vi "read pre-execution timing tags.vi"(8 "error in":errorcluster, 11 "Standard Engine Configuration in":refnum<class "Standard Engine Configuration.lvclass">) -> (0 "error out":errorcluster, 2 "execution timing tags":T1, 3 "Standard Engine Configuration out":refnum<class "Standard Engine Configuration.lvclass">)   [LabVIEW 2013, in "Standard Engine Configuration.lvclass"]
doc: "Returns the timing status tags previously configured by the 'enable timing reporting.vi'."
uses:
  Standard Engine Configuration.lvclass
  execution timing tags.ctl
  Standard Engine Configuration.lvclass/Standard Engine Configuration.ctl
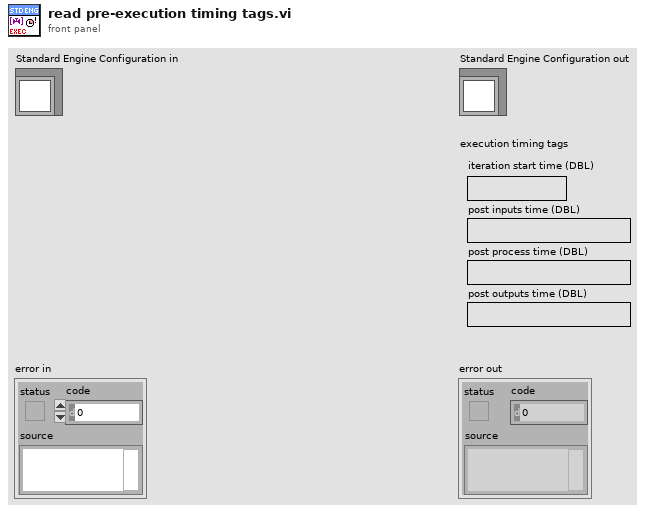
[diagram p1: front panel]
types:
  T1 = typedef "Standard Engine Configuration.lvclass/execution timing tags.ctl" = cluster{"iteration start time (DBL)":string, "post inputs time (DBL)":string, "post process time (DBL)":string, "post outputs time (DBL)":string}
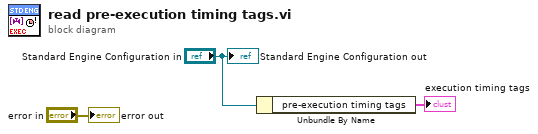
[diagram p0: block diagram]
diagram:
  n1 = Unbundle By Name("Standard Engine Configuration in") -> ("pre-execution timing tags"=→"execution timing tags":T1)
  "error out" <- "error in"
  "Standard Engine Configuration out" <- "Standard Engine Configuration in"
